vi "Run Bfr Rx - Cached - Copy Flush Add.vi"(4 "Data Size in":u64, 5 "Cache Buffer":u64 format="%016x", 6 "Copy and Flush":bool, 7 "External Buffer":u64 format="%016x", 8 "error in (no error)":errorcluster, 9 "Null Data in":u8[](array[numeric]), 10 "Data in":u8[](array[numeric]), 11 "Data Offset in":u64) -> (0 "error out":errorcluster, 3 "Data Offset out":u64)   [LabVIEW 2021, in "UDP-Custom-Device Engine.lvlib"]
uses:
  UDP-Custom-Device Engine.lvlib
  <vilib>/NI VeriStand/VeriStand Data/Pointer Operations/Pointer.In-Place Read.vi
  <vilib>/NI VeriStand/VeriStand Data/Pointer Operations/Pointer.In-Place Read (1D U8).vi
  <vilib>/NI VeriStand/VeriStand Data/Pointer Operations/Pointer.Write.vi
  <vilib>/NI VeriStand/VeriStand Data/Pointer Operations/Pointer.Write (1D U8).vi
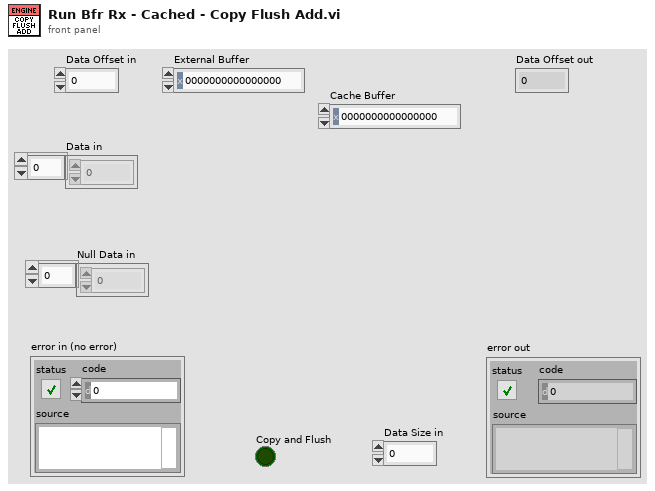
[diagram p1: front panel]
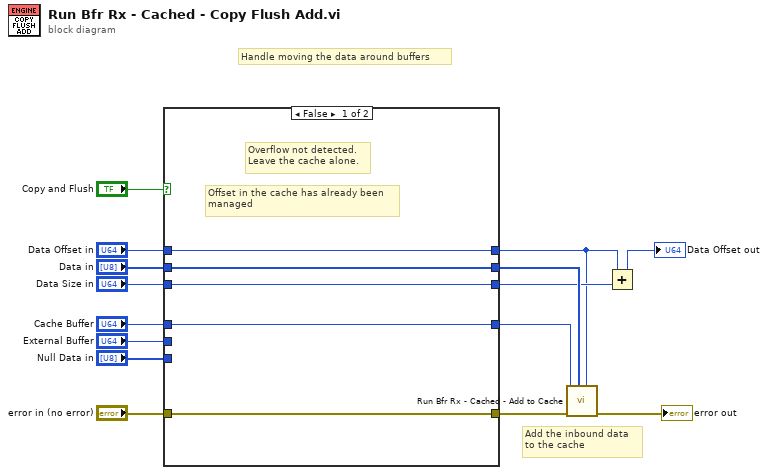
[diagram p0: block diagram]
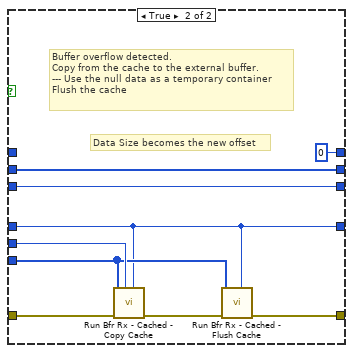
[diagram p2: hidden frame]
diagram:
  # "Add the inbound data\nto the cache"
  # "Handle moving the data around buffers"
  n1 = case shown="False" "Copy and Flush" {
    tunnel: [w20 w23] -> w4
    tunnel: "error in (no error)" -> [w20 w29]
    tunnel: "External Buffer" -> [_ w28]
    tunnel: "Data Offset in" -> [w19 _]
    tunnel: "Data Size in" -> [w16 w21]
    tunnel: "Data in" -> [w18 w27]
    tunnel: "Null Data in" -> [_ w26]
    tunnel: "Cache Buffer" -> [w17 w25]
    tunnel: [w19 u64 0 ("Data Size in")] -> w1
    tunnel: [w18 w27] -> w6
    tunnel: [w17 w25] -> w7
    tunnel: [w16 w21] -> w3
    frame False {
      # "Offset in the cache has already been\nmanaged"
      # "Overflow not detected.\nLeave the cache alone."
    }
    frame True {
      # "Data Size becomes the new offset"
      # "Buffer overflow detected.\nCopy from the cache to the external buffer.\n--- Use the null data as a temporary container\nFlush the cache"
      n2 = call "Run Bfr Rx - Cached - Copy Cache.vi"("Cache Buffer"=w25, "External Buffer"=w28, "error in (no error)"=w29, "Temp Data in"=w26) -> ("error out"=w24:errorcluster)  [unwired: 7 in]
      n3 = call "Run Bfr Rx - Cached - Flush Cache.vi"("Cache Buffer"=w25, "error in (no error)"=w24, "Null Data in"=w26) -> ("error out"=w23:errorcluster)  [unwired: 8 in]
    }
  }
  n4 = call "Run Bfr Rx - Cached - Add to Cache.vi"("Data Offset in"=w1, "Data in"=w6, "error in (no error)"=w4, "Cache Buffer"=w7) -> ("error out"=→"error out":errorcluster)  [unwired: 7 in]
  n5 = Add(x=w1, y=w3) -> (x+y=→"Data Offset out":u64)
